vi "Creators Creator Queue Alias.vi"(11 "TEMPLATE Event in":refnum<class "TEMPLATE Event.lvclass">) -> (2 "Creator Queue Alias":string, 3 "TEMPLATE Event out":refnum<class "TEMPLATE Event.lvclass">)   [LabVIEW 2021, in "_Template.lvlib" / "Templates.lvlib" / "TEM Event.lvlib" / "TEMPLATE Event.lvclass"]
uses:
  TEMPLATE Event.lvclass
  TEMPLATE Event.lvclass/TEMPLATE Event.ctl
  <vilib>/Nathan Davis/jettl/jettl/Event/Event.lvclass
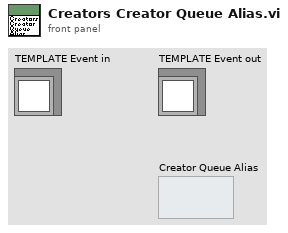
[diagram p1: front panel]
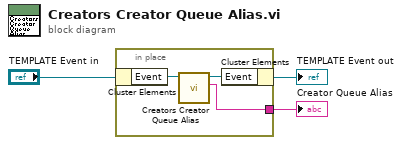
[diagram p0: block diagram]
diagram:
  n1 = in-place {
    in-place-border: [w4] -> w1
    n2 = in-place-cluster #1("TEMPLATE Event in") -> ("Event"=w6:refnum<class "Event.lvclass">)
    n3 = call-dynamic "Creators Creator Queue Alias.vi"("Event in"=w6) -> ("Creator Queue Alias"=w4:string, "Event out"=w5:refnum<class "Event.lvclass">)  [unwired: 9 in]
    n4 = in-place-cluster #1("Event"=w5) -> (→"TEMPLATE Event out":refnum<class "TEMPLATE Event.lvclass">)
  }
  "Creator Queue Alias" <- w1
